vi "Append CSM AppDir If Relative.vi"(4 "Relative Path (.)":path=path "") -> (1 "Application Directory (+ Relative)":path)   [LabVIEW 2017, in "CSM File Logger.lvlib"]
uses:
  CSM File Logger.lvlib
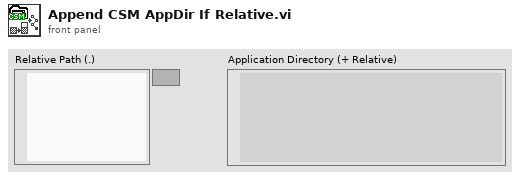
[diagram p1: front panel]
types:
  T1 = enum16{"Absolute path", "Relative path", "<Not A Path>"}
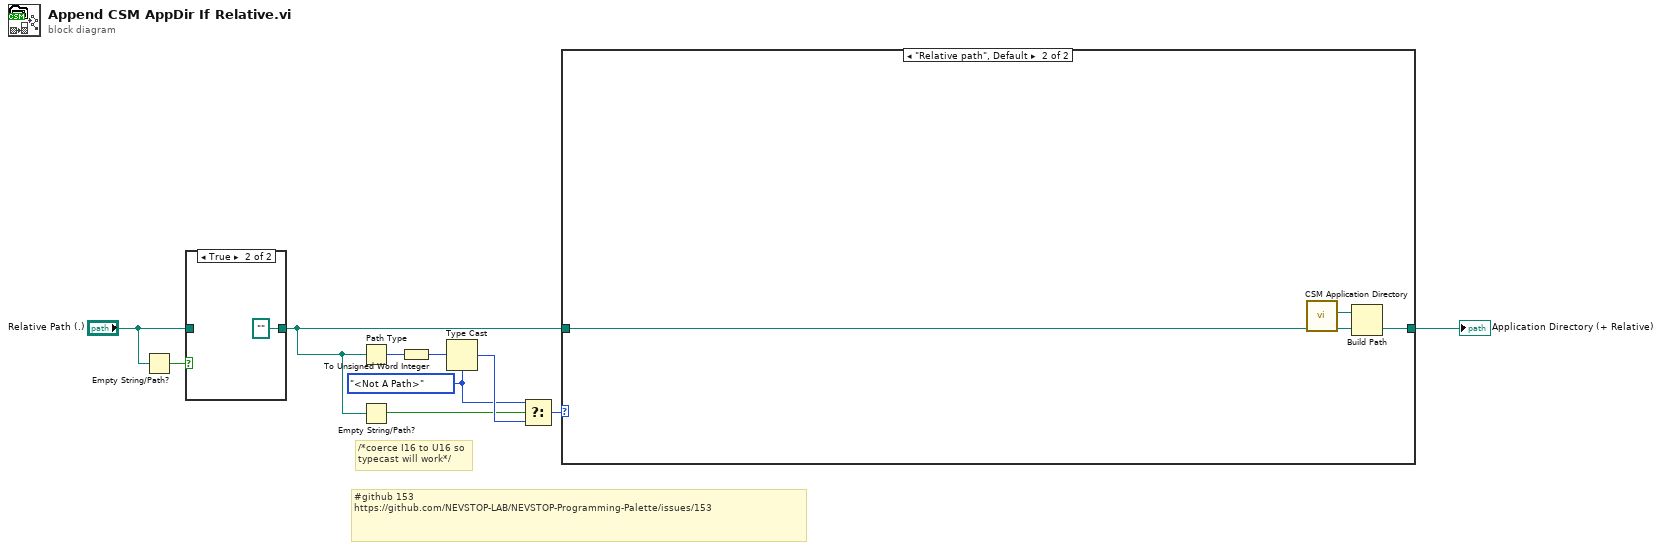
[diagram p0: block diagram]
diagram:
  w3 = T1."<Not A Path>"
  # "/*coerce I16 to U16 so typecast will work*/"
  # "#github 153\nhttps://github.com/NEVSTOP-LAB/NEVSTOP-Programming-Palette/issues/153"
  n1 = Empty String/Path?(string/path="Relative Path (.)") -> (empty?=w8:bool)
  n2 = case shown="True" w8 {
    tunnel: [w11 path "" ("Relative path (.)")] -> w7
    tunnel: "Relative Path (.)" -> [w11 _]
    frame False {
    }
    frame True {
    }
  }
  n3 = Path Type(1:w7) -> (0:w1:i16)
  n4 = Empty String/Path?(string/path=w7) -> (empty?=w2:bool)
  n5 = To Unsigned Word Integer(number=w1) -> (unsigned 16bit integer=w5:u16)
  n6 = Type Cast(type=w3, x=w5) -> (*(type *) &x=w4:T1)
  n7 = Select(t=w3, s=w2, f=w4) -> (s? t:f=w9:T1)
  n8 = case shown="\"Relative path\", Default" w9 {
    tunnel: [w13 w16] -> w10
    tunnel: w7 -> [w13 w15]
    frame "Absolute path" {
    }
    frame "Relative path", Default {
      n9 = call "CSM Application Directory.vi"() -> ("CSM Application Dir"=w14:path)  [unwired: 11 in]
      n10 = Build Path(base path=w14, name or relative path=w15) -> (appended path=w16:path)
    }
  }
  "Application Directory (+ Relative)" <- w10
